vi "FV_get_move.vi"(8 "error in":errorcluster, 11 "VISA":refnum<visa-resource-name>) -> (0 "error out":errorcluster, 1 "status":bool, 2 "step":i32, 3 "VISA out":refnum<visa-resource-name>)   [LabVIEW 2019]
panel:
  out "return count":u32
  out "read buffer":string
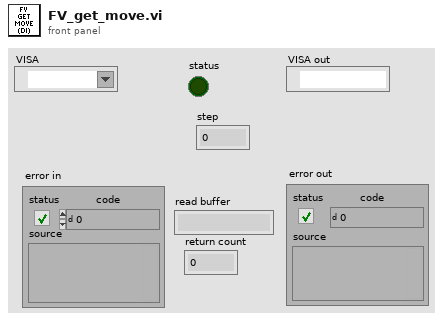
[diagram p1: front panel]
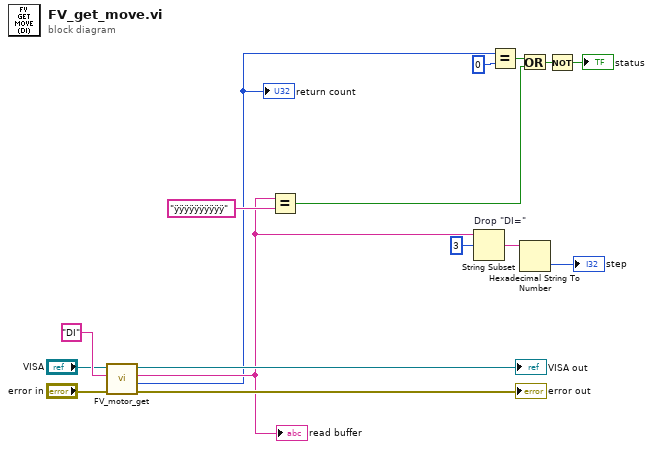
[diagram p0: block diagram]
diagram:
  n1 = call "FV_motor_get.vi"("error in"="error in", "command"="DI", "VISA in"="VISA") -> ("error out"=→"error out":errorcluster, "ret_bytes"=w1:u32, "return"=w2:string, "VISA out"=→"VISA out":refnum<visa-resource-name>)  [unwired: 5 in]
  "read buffer" <- w2
  "return count" <- w1
  n2 = Equal?(x=w2, y="ÿÿÿÿÿÿÿÿÿÿ") -> (x = y?=w7:bool)
  n3 = String Subset "Drop \"DI=\""(string=w2, offset (0)=3) -> (substring=w12:string)  [unwired: 1 in]
  n4 = Equal?(x=w1, y=u32 0) -> (x = y?=w8:bool)
  n5 = Or(x=w8, y=w7) -> (x .or. y?=w6:bool)
  n6 = Hexadecimal String To Number(string=w12) -> (number=→"step":u32)  [unwired: 2 in, 1 out]
  n7 = Not(x=w6) -> (.not. x?=→"status":bool)
